vi "Get AccessType+.vi"(8 "Error In":errorcluster, 11 "reference in":refnum<class "OD Entry.lvclass">) -> (0 "Error Out":errorcluster, 1 "Defined?":bool, 2 "AccessType":T1=enum."const", 3 "reference out":refnum<class "OD Entry.lvclass">)   [LabVIEW 2019, in "Electronic Datasheet.lvlib" / "OD Entry.lvclass"]
uses:
  OD Entry.lvclass
  OD Sub-Entry/OD Sub-Entry.lvclass
  Object Type/Object Type Base.lvclass
  Access Type.ctl
  Electronic Datasheet.lvlib
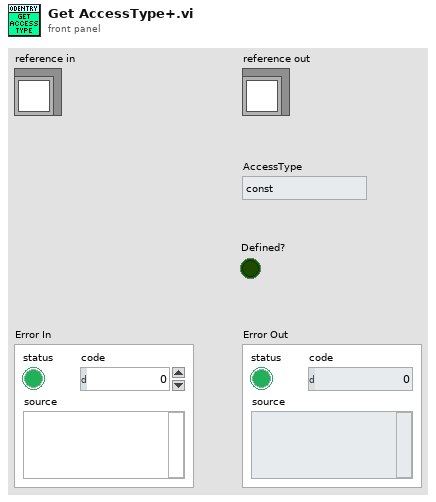
[diagram p1: front panel]
types:
  T1 = typedef "Electronic Datasheet.lvlib/Access Type.ctl" = enum16{"ro", "wo", "rw", "rwr", "rww", "const"}
  T2 = typedef "Electronic Datasheet.lvlib/OD Entry.lvclass/ObjectAttributes.ctl" = cluster{"Index":u16, "ObjectType":refnum<class "Object Type Base.lvclass">, "Denotation":string, "Count":u8, "ObjExtend":u8, "Label":string, "Description":string, "PDO Mapping Type":T3, "Sub-Entries":map{u8, refnum<class "OD Sub-Entry.lvclass">}}
  T3 = typedef "Electronic Datasheet.lvlib/PDO Mapping Type.ctl" = enum16{"no", "optional", "RPDO", "TPDO", "UNKNOWN"}
  T4 = typedef "Electronic Datasheet.lvlib/Object Type.ctl" = u8
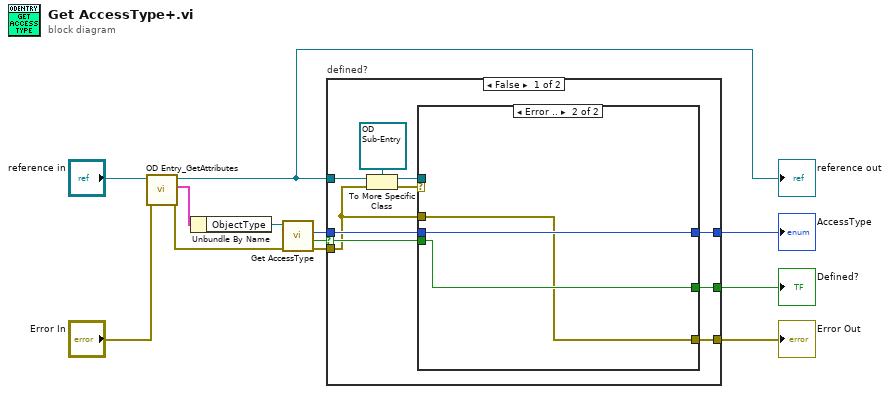
[diagram p0: block diagram]
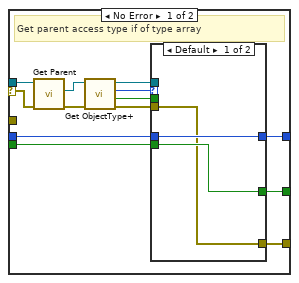
[diagram p2: hidden frame]
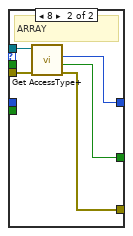
[diagram p3: hidden frame]
diagram:
  n1 = call "OD Entry_GetAttributes.vi"("Error In"="Error In", "reference in"="reference in") -> ("Error Out"=w8:errorcluster, "Data"=w10:T2, "reference out"=w1:refnum<class "OD Entry.lvclass">)  [unwired: 6 in, 1 out]
  "reference out" <- w1
  n2 = Unbundle By Name(w10) -> ("ObjectType"=w9:refnum<class "Object Type Base.lvclass">)
  n3 = call-dynamic "Get AccessType.vi"("error in"=w8, "Object Type in"=w9) -> ("error out"=w6:errorcluster, "Defined?"=w7:bool, "AccessType"=w5:T1)  [unwired: 6 in, 1 out]
  n4 = case "defined?" shown="False" w7 {
    selector: w7 -> [w15 w48]
    tunnel: w1 -> [w14 _]
    tunnel: w6 -> [w13 w47]
    tunnel: w5 -> [w16 w49]
    tunnel: [w17 w49] -> w4
    tunnel: [w18 w48] -> w3
    tunnel: [w19 w47] -> w2
    frame False {
      n5 = To More Specific Class(target class=refnum<class "OD Sub-Entry.lvclass"> refnum ("sub entry"), reference=w14, error in=w13) -> (specific class reference=w22:refnum<class "OD Sub-Entry.lvclass">, error out=w20:errorcluster)
      n6 = case shown="Error .." w20 {
        selector: w20 -> [w34 _]
        tunnel: w22 -> [w35 _]
        tunnel: [w28 w44] -> w19
        tunnel: [w27 w46] -> w18
        tunnel: [w25 w45] -> w17
        tunnel: w16 -> [w26 w45]
        tunnel: w15 -> [w24 w46]
        tunnel: w13 -> [_ w44]
        frame No Error {
          # "Get parent access type if of type array"
          n7 = call "Get Parent.vi"("Error In"=w34, "reference in"=w35) -> ("Error Out"=w33:errorcluster, "Parent"=w32:refnum<class "OD Entry.lvclass">)  [unwired: 7 in, 1 out]
          n8 = call "Get ObjectType+.vi"("Error In"=w33, "reference in"=w32) -> ("Error Out"=w29:errorcluster, "Defined?"=w30:bool, "ObjectType"=w31:T4, "reference out"=w23:refnum<class "OD Entry.lvclass">)  [unwired: 6 in]
          n9 = case shown="Default" w31 {
            tunnel: w30 -> [_ _]
            tunnel: w29 -> [w36 w42]
            tunnel: [w36 w41] -> w28
            tunnel: [w37 w40] -> w27
            tunnel: w26 -> [w38 _]
            tunnel: [w38 w39] -> w25
            tunnel: w24 -> [w37 _]
            tunnel: w23 -> [_ w43]
            frame Default {
            }
            frame 8 {
              # "ARRAY"
              n10 = call "Get AccessType+.vi"("Error In"=w42, "reference in"=w43) -> ("Error Out"=w41:errorcluster, "Defined?"=w40:bool, "AccessType"=w39:T1)  [unwired: 6 in, 1 out]
            }
          }
        }
        frame Error {
        }
      }
    }
    frame True {
    }
  }
  "Error Out" <- w2
  "AccessType" <- w4
  "Defined?" <- w3
